vi "Set state DSP402.vi"(4 "error in (no error)":errorcluster, 6 "State":T1, 7 "DSP402 in":refnum<class "DSP402.lvclass">) -> (0 "error out":errorcluster, 3 "DSP402 out":refnum<class "DSP402.lvclass">)   [LabVIEW 2017, in "canopen.lvlib" / "DSP402.lvclass"]
uses:
  DSP402.lvclass
  DriveState.ctl
  DSP402.lvclass/DSP402.ctl
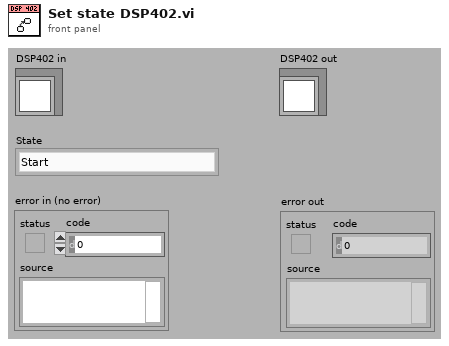
[diagram p1: front panel]
types:
  T1 = typedef "canopen.lvlib/DSP402.lvclass/DriveState.ctl" = enum16{"Start", "Not ready to switch on", "Switch on disabled", "Ready to switch on", "Switched on", "Operation enable", "Fault reaction active", "Fault", "Quick stop active"}
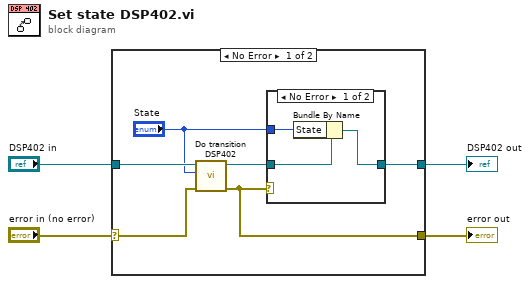
[diagram p0: block diagram]
diagram:
  n1 = case shown="No Error" "error in (no error)" {
    selector: "error in (no error)" -> [w6 w15]
    tunnel: "DSP402 in" -> [w10 w16]
    tunnel: [w9 w16] -> w3
    tunnel: [w7 w15] -> w2
    frame No Error {
      n2 = call "Do transition DSP402.vi"("error in (no error)"=w6, "State"="State", "DSP402 in"=w10) -> ("error out"=w7:errorcluster, "DSP402 out"=w8:refnum<class "DSP402.lvclass">)  [unwired: 3 out]
      n3 = case shown="No Error" w7 {
        tunnel: [w12 w14] -> w9
        tunnel: w8 -> [w13 w14]
        tunnel: "State" -> [w11 _]
        frame No Error {
          n4 = Bundle By Name(cluster=w13, "State"=w11) -> (w12:refnum<class "DSP402.lvclass">)
        }
        frame Error {
        }
      }
    }
    frame Error {
    }
  }
  "error out" <- w2
  "DSP402 out" <- w3
